vi "array_for_overlay.vi"(11 "Array in":dbl[][](array[numeric])) -> (3 "Array out":cluster{"X":i32, "Y":i32}[](array[cluster]))   [LabVIEW 2017]
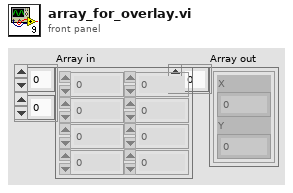
[diagram p1: front panel]
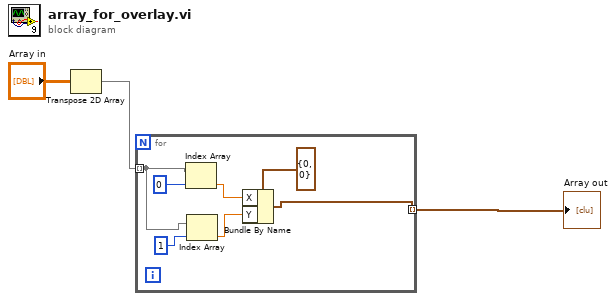
[diagram p0: block diagram]
diagram:
  n1 = Transpose 2D Array(2D array="Array in") -> (transposed array=w1:dbl[][])
  n2 = for {
    tunnel: w1 -> [w9] mode=indexing
    tunnel: [w4] -> w3 mode=indexing
    n3 = Index Array(array=w9, index=0) -> (element=w6:dbl)
    n4 = Index Array(array=w9, index=1) -> (element=w5:dbl)
    n5 = Bundle By Name(cluster=cluster{"X":i32, "Y":i32} {"X"=0, "Y"=0} ("Point"), "X"=w6, "Y"=w5) -> (w4:cluster{"X":i32, "Y":i32})
  }
  "Array out" <- w3
